vi "initilize Hioky.vi"(8 "error in (no error)":errorcluster, 9 "Serial Configuration":T1={"Baud Rate"=9600, "Parity"=0, "Data Bits"=8} {"Data Bits" items=["7"=7, "8"=8]; "Parity" items=["None", "Odd", "Even"]; "Baud Rate" items=["300"=300, "600"=600, "1200"=1200, "2400"=2400, "4800"=4800, "9600"=9600, "19200"=19200]}, 11 "VISA resource name":refnum<visa-resource-name>) -> (0 "error out":errorcluster, 3 "VISA resource name out":refnum<visa-resource-name>)   [LabVIEW 2017]
uses:
  <vilib>/Instr/_visa.llb/VISA Flush IO Buffer Mask.ctl
  <instrlib>/Agilent 34401/Agilent 34401.lvlib
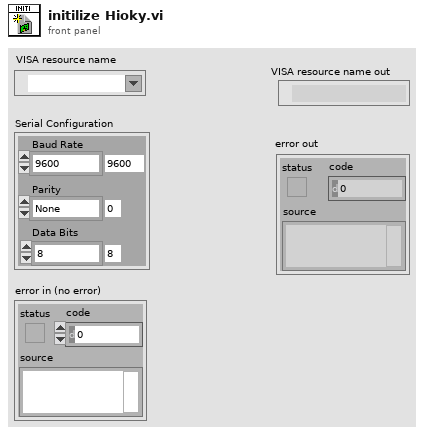
[diagram p1: front panel]
types:
  T1 = cluster{"Baud Rate":u32, "Parity":u16, "Data Bits":u16}
  T2 = typedef "VISA Flush IO Buffer Mask.ctl" = u16
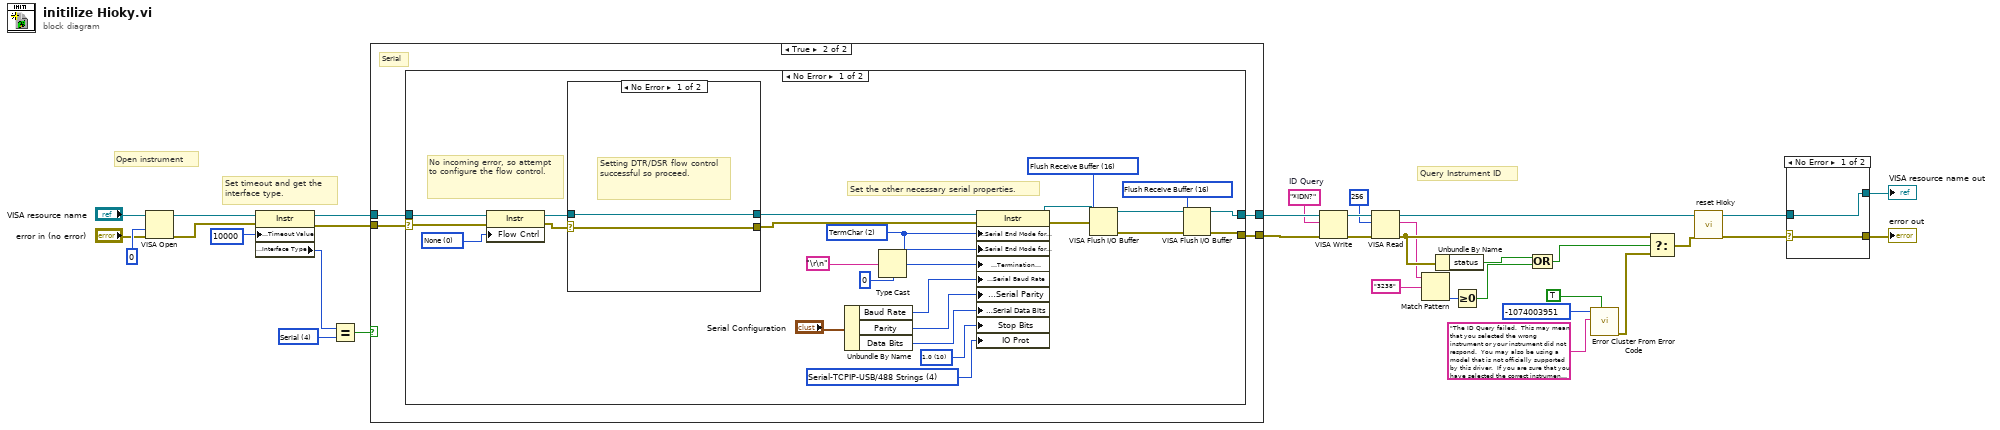
[diagram p0: block diagram]
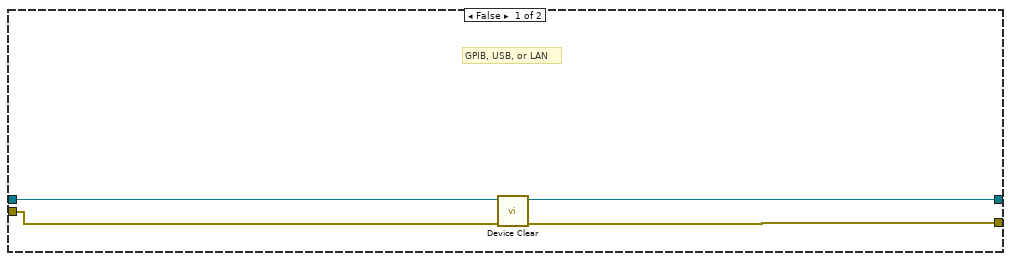
[diagram p2: hidden frame]
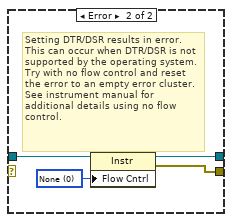
[diagram p3: hidden frame]
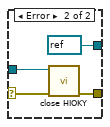
[diagram p5: hidden frame]
diagram:
  w11 = "*IDN?"  # ID Query
  w25 = u16 4 items=["GPIB"=1, "VXI"=2, "GPIB-VXI"=3, "Serial"=4, "PXI"=5, "TCPIP"=6, "USB"=7] ("Interface Information:Interface Type")
  # "Set timeout and get the\ninterface type."
  # "Query Instrument ID"
  # "Open instrument"
  n1 = VISA Open(access mode=u32 0, error in (no error)="error in (no error)", VISA resource name="VISA resource name") -> (VISA resource name=w31:refnum<visa-resource-name>, error out=w32:errorcluster)  [unwired: 2 in]
  n2 = property on="Property Node" class="Instr"(reference=w31, error in=w32, "General Settings:Timeout Value"=u32 10000) -> (reference out=w33:refnum<visa-resource-name>, error out=w34:errorcluster, "Interface Information:Interface Type"=w22:u16)
  n3 = Equal?(x=w22, y=w25) -> (x = y?=w24:bool)
  n4 = case shown="True" w24 {
    tunnel: [w36 w42] -> w28
    tunnel: [w35 w41] -> w30
    tunnel: w33 -> [w37 w40]
    tunnel: w34 -> [w38 w39]
    frame False {
      # "GPIB, USB, or LAN"
      n5 = call <instrlib>:"Device Clear.vi"("error in (no error)"=w38, "VISA Resource Name"=w37) -> ("error out"=w35:errorcluster, "VISA Resource Out"=w36:refnum<visa-resource-name>)  [unwired: 8 in]
    }
    frame True {
      # "Serial"
      n6 = case shown="No Error" w39 {
        selector: w39 -> [w52 w74]
        tunnel: [w47 w75] -> w42
        tunnel: [w46 w74] -> w41
        tunnel: w40 -> [w66 w75]
        frame No Error {
          w49 = T2 16 items=["Flush Receive Buffer"=16, "Write Transmit Buffer to Device"=32, "Flush Receive Buffer (No I/O)"=64, "Flush Transmit Buffer"=128] ("Mask")
          w50 = T2 16 items=["Flush Receive Buffer"=16, "Write Transmit Buffer to Device"=32, "Flush Receive Buffer (No I/O)"=64, "Flush Transmit Buffer"=128] ("Mask")
          w63 = u16 4 items=["Normal"=1, "VXI/FDC"=2, "GPIB/HS488"=3, "Serial-TCPIP-USB/488 Strings"=4, "USBTMC/Vendor-Specific"=5] ("Message Based Settings:IO Protocol")
          w62 = u16 10 items=["1.0"=10, "1.5"=15, "2.0"=20] ("Serial Settings:Serial Stop Bits")
          w56 = u16 2 items=["None", "LastBit", "TermChar"] ("Serial Settings:Serial End Mode for Reads")
          w67 = u16 0 items=["None", "XON/XOFF", "RTS/CTS", "XON/XOFF & RTS/CTS", "DTR/DSR", "XON/XOFF & DTR/DSR"] ("Serial Settings:Serial Flow Control")
          # "Set the other necessary serial properties."
          # "No incoming error, so attempt to configure the flow control."
          n7 = property on="Property Node" class="Instr"(reference=w66, error in=w52, "Flow Cntrl"=w67) -> (reference out=w65:refnum<visa-resource-name>, error out=w64:errorcluster)
          n8 = case shown="No Error" w64 {
            selector: w64 -> [w68 _]
            tunnel: w65 -> [w69 w70]
            tunnel: [w69 w71] -> w53
            tunnel: [w68 w72] -> w54
            frame No Error {
              # "Setting DTR/DSR flow control successful so proceed."
            }
            frame Error {
              w73 = u16 0 items=["None", "XON/XOFF", "RTS/CTS", "XON/XOFF & RTS/CTS", "DTR/DSR", "XON/XOFF & DTR/DSR"] ("Serial Settings:Serial Flow Control")
              # "Setting DTR/DSR results in error. This can occur when DTR/DSR is not supported by the operating system.  Try with no flow control and reset the error to an empty error cluster. See instrument manual for additional details using no flow control."
              n9 = property on="Property Node" class="Instr"(reference=w70, "Flow Cntrl"=w73) -> (reference out=w71:refnum<visa-resource-name>, error out=w72:errorcluster)  [unwired: 1 in]
            }
          }
          n10 = Unbundle By Name("Serial Configuration") -> ("Baud Rate"=w59:u32, "Parity"=w61:u16, "Data Bits"=w60:u16)
          n11 = Type Cast(type=u8 0, x="\r\n") -> (*(type *) &x=w57:u8)
          n12 = property on="Property Node" class="Instr"(reference=w53, error in=w54, "Serial Settings:Serial End Mode for Reads"=w56, "Serial Settings:Serial End Mode for Writes"=w56, "Message Based Settings:Termination Character"=w57, "Serial Settings:Serial Baud Rate"=w59, "Serial Settings:Serial Parity"=w61, "Serial Settings:Serial Data Bits"=w60, "Stop Bits"=w62, "IO Prot"=w63) -> (reference out=w43:refnum<visa-resource-name>, error out=w44:errorcluster)
          n13 = VISA Flush I/O Buffer(VISA resource name=w43, mask (16)=w50, error in (no error)=w44) -> (VISA resource name out=w48:refnum<visa-resource-name>, error out=w45:errorcluster)
          n14 = VISA Flush I/O Buffer(VISA resource name=w48, mask (16)=w49, error in (no error)=w45) -> (VISA resource name out=w47:refnum<visa-resource-name>, error out=w46:errorcluster)
        }
        frame Error {
          # "If there is an error in, do not attempt to set additional serial parameters."
        }
      }
    }
  }
  n15 = VISA Write(VISA resource name=w28, write buffer=w11, error in (no error)=w30) -> (VISA resource name out=w15:refnum<visa-resource-name>, error out=w14:errorcluster)  [unwired: 1 out]
  n16 = VISA Read(VISA resource name=w15, byte count=u32 256, error in (no error)=w14) -> (VISA resource name out=w17:refnum<visa-resource-name>, read buffer=w1:string, error out=w5:errorcluster)  [unwired: 1 out]
  n17 = Match Pattern(string=w1, regular expression="3238") -> (offset past match=w6:i32)  [unwired: 1 in, 3 out]
  n18 = Unbundle By Name(w5) -> ("status"=w4:bool)
  n19 = Greater Or Equal To 0?(x=w6) -> (x >= 0?=w3:bool)
  n20 = Compound Arithmetic op=OR(w4, w3) -> (w2:bool)
  n21 = call <vilib>:"Error Cluster From Error Code.vi"("show call chain? (False)"=TRUE, "error message (\"\")"="The ID Query failed.  This may mean that you selected the wrong instrument or your instrument did not respond.  You may also be using a model that is not officially supported by this driver.  If you are sure that you have selected the correct instrument and it is responding, try disabling the ID Query." ("Source (VI Name)"), "error code (0)"=-1074003951 ("Code")) -> ("error out"=w10:errorcluster)  [unwired: 6 in]
  n22 = Select(t=w5, s=w2, f=w10) -> (s? t:f=w16:errorcluster)
  n23 = call "reset Hioky.vi"("error in (no error)"=w16, "VISA resource name"=w17) -> ("error out"=w18:errorcluster, "VISA resource name out"=w19:refnum<visa-resource-name>)  [unwired: 8 in]
  n24 = case shown="No Error" w18 {
    selector: w18 -> [w77 w79]
    tunnel: [w76 refnum<visa-resource-name> refnum ("VISA resource name out")] -> w27
    tunnel: [w77 w78] -> w29
    tunnel: w19 -> [w76 w80]
    frame No Error {
    }
    frame Error {
      n25 = call "close HIOKY.vi"("error in (no error)"=w79, "VISA resource name"=w80) -> ("error out"=w78:errorcluster)  [unwired: 9 in]
    }
  }
  "VISA resource name out" <- w27
  "error out" <- w29
